vi "write4Byte Tx Only.vi"(6 "data":u32, 7 "address":u16, 9 "id":u8, 10 "protocol_version":i32, 11 "port_num":i32) -> ()   [LabVIEW 2021, in "dxl_x86_c.lvlib"]
doc: "WINDECLSPEC void write4ByteTxOnly (int port_num, int protocol_version, uint8_t id, uint16_t address, uint32_t data);"
uses:
  dxl_x86_c.lvlib
  dxl_x86_c.dll
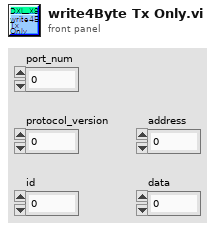
[diagram p1: front panel]
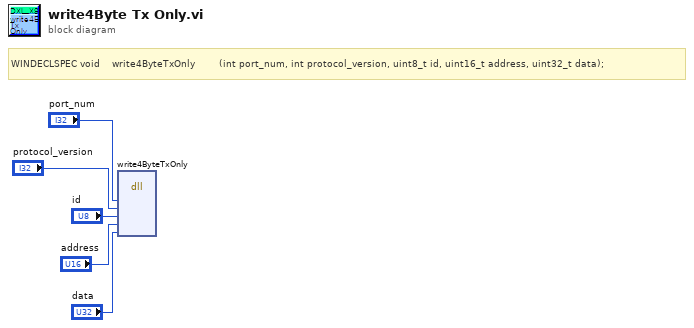
[diagram p0: block diagram]
diagram:
  # "WINDECLSPEC void    write4ByteTxOnly        (int port_num, int protocol_version, uint8_t id, uint16_t address, uint32_t data);"
  n1 = dll-call lib="C:/Users/ashek/Desktop/ashekim/ws/DynamixelSDK/labview/labview/dxl_x86_c.*" fn="write4ByteTxOnly"("port_num"="port_num", "protocol_version"="protocol_version", "id"="id", "address"="address", "data"="data") -> ()  [unwired: 9 in, 2 out]
